vi "Parse Element.vi"(0 "queue in":refnum<queue>, 3 "error in (no error)":errorcluster) -> (14 "queue out":refnum<queue>, 15 "State":string, 16 "Arg":string, 17 "Data":variant)   [LabVIEW 2023, in "FaKI State Machine.lvlib"]
doc: "Parses the queue and outputs the next state, along with its associated argument and data if they exist. If <B>error in</B> contains an error, the \"Error Handler\" state will the output."
uses:
  FaKI State Machine.lvlib
  <vilib>/Utility/error.llb/Trim Whitespace One-Sided.vi
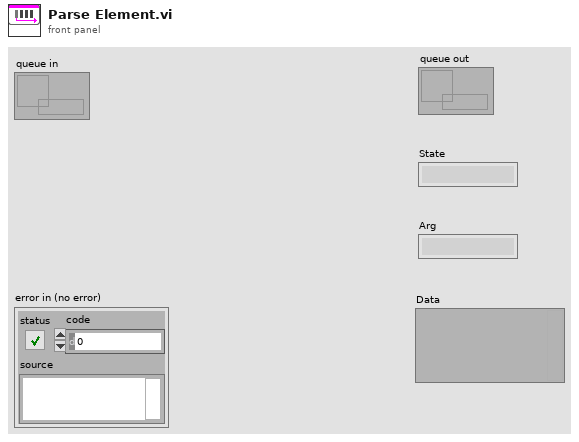
[diagram p1: front panel]
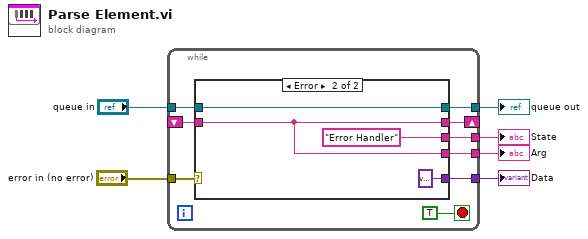
[diagram p0: block diagram]
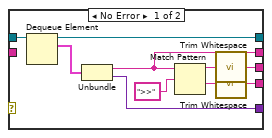
[diagram p2: hidden frame]
diagram:
  n1 = while {
    tunnel: "error in (no error)" -> [w15]
    tunnel: [w14] -> w5
    tunnel: [w13] -> w4
    tunnel: [w12] -> w3
    shift-right: [w8] -> _
    shift-left: _ -> [w7]
    tunnel: "queue in" -> [w11]
    tunnel: [w10] -> w1
    stop <- TRUE stop-if-true
    n2 = case shown="Error" w15 {
      tunnel: [w22 variant] -> w13
      tunnel: [w21 w26] -> w12
      tunnel: [w20 "Error Handler" ("trimmed string")] -> w14
      tunnel: w11 -> [w19 w27]
      tunnel: [w17 w27] -> w10
      tunnel: [w16 w26] -> w8
      tunnel: w7 -> [_ w26]
      frame No Error {
        n3 = Dequeue Element(queue=w19) -> (queue out=w17:refnum<queue>, element=w18:cluster{string, variant})  [unwired: 2 in, 2 out]
        n4 = Unbundle(w18) -> (w16:string, w22:variant)
        n5 = Match Pattern(string=w16, regular expression=">>") -> (before substring=w24:string, after substring=w23:string)  [unwired: 1 in, 2 out]
        n6 = call <vilib>:"Trim Whitespace.vi"("string"=w24) -> ("trimmed string"=w20:string)  [unwired: 1 in]
        n7 = call <vilib>:"Trim Whitespace.vi"("string"=w23) -> ("trimmed string"=w21:string)  [unwired: 1 in]
      }
      frame Error {
      }
    }
  }
  "State" <- w5
  "Data" <- w4
  "Arg" <- w3
  "queue out" <- w1
